vi "UpdateApp.vi"(7 "DefaultAppConfig? (f)":bool, 8 "ErrorArray In":errorcluster[](array[cluster]), 10 "clBusData in":T1={"BusNumber"=0, "EvtPluginINIFilePath"=path "", "EvtParams"=[], "EvtConfig"={"UTC Time 0"=timestamp(0 s since 1904-01-01), "Nominal Frequency"=60, "Reporting Rate"=60, "Fsamp"=960, "PosSeq"=FALSE}, "Start Time"=0.0, "End Time"=0.0, "PmuImpairPluginINIFilePath"=path "", "PmuImpairParams "=[["960"], ["8.19"], ["164"]], "PmuImpairConfig"={"FilterType"="", "bPosSeq"=TRUE}, "NetImpPluginINIFilePath"=path "", "NetImpParams"=[], "FlagImpPluginINIFilePath"=path "", "FlagImpParams"=[], "EvtReportArray"=[], "EventSignalArray"=[], "ImpairReportArray"=[], "NetworkTime"=[], "PktLoss"=[], "FlagImpArray"=[], "OutputToFilePluginINIFilePath"=path "", "Output File Path"=path "", "clConfigOptions"={"TIME_BASE"=1000000, "STN"="Bus_1", "IDCODE"=0, "rdoPolRect"=enum."Rectangular", "rdoFloatInt"=enum."Float", "PHUNIT"=1000000, "rdoFreqDfreq"=enum."Float", "CHNAM"=["VA", "VB", "VC", "V+", "IA", "IB", "IC", "I+"], "chkCfg2Prefix"=TRUE}, "AppPluginINIFilePath"=path "", "AppConfig"=variant, "AppOutput"=variant} {"clConfigOptions"."PHUNIT" max=16777216 step=1 format="%08d"; "clConfigOptions"."IDCODE" format="%02x"; "clConfigOptions"."TIME_BASE" max=16777216 step=1 format="%08d"; "ImpairReportArray"."Synx" format="%#_4g"; "EvtReportArray"."Synx" format="%#_4g"; "EvtConfig"."Reporting Rate" items=["10 FPS"=10, "12 FPS"=12, "15 FPS"=15, "20 FPS"=20, "25 FPS"=25, "30 FPS"=30, "50 FPS"=50, "60 FPS"=60]; "EvtConfig"."Nominal Frequency" items=["50 Hz"=50, "60 Hz"=60]}, 11 "Bus.lvclass":refnum<class "Bus.lvclass">) -> (0 "ErrorArray Out":errorcluster[](array[cluster]), 2 "clBusData out":T1={"BusNumber"=0, "EvtPluginINIFilePath"=path "", "EvtParams"=[], "EvtConfig"={"UTC Time 0"=timestamp(0 s since 1904-01-01), "Nominal Frequency"=60, "Reporting Rate"=60, "Fsamp"=960, "PosSeq"=FALSE}, "Start Time"=0.0, "End Time"=0.0, "PmuImpairPluginINIFilePath"=path "", "PmuImpairParams "=[["960"], ["8.19"], ["164"]], "PmuImpairConfig"={"FilterType"="", "bPosSeq"=TRUE}, "NetImpPluginINIFilePath"=path "", "NetImpParams"=[], "FlagImpPluginINIFilePath"=path "", "FlagImpParams"=[], "EvtReportArray"=[], "EventSignalArray"=[], "ImpairReportArray"=[], "NetworkTime"=[], "PktLoss"=[], "FlagImpArray"=[], "OutputToFilePluginINIFilePath"=path "", "Output File Path"=path "", "clConfigOptions"={"TIME_BASE"=1000000, "STN"="Bus_1", "IDCODE"=0, "rdoPolRect"=enum."Rectangular", "rdoFloatInt"=enum."Float", "PHUNIT"=1000000, "rdoFreqDfreq"=enum."Float", "CHNAM"=["VA", "VB", "VC", "V+", "IA", "IB", "IC", "I+"], "chkCfg2Prefix"=TRUE}, "AppPluginINIFilePath"=path "", "AppConfig"=variant, "AppOutput"=variant} {"clConfigOptions"."PHUNIT" max=16777216 step=1 format="%08d"; "clConfigOptions"."IDCODE" format="%02x"; "clConfigOptions"."TIME_BASE" max=16777216 step=1 format="%08d"; "ImpairReportArray"."Synx" format="%#_4g"; "EvtReportArray"."Synx" format="%#_4g"; "EvtConfig"."Reporting Rate" items=["10 FPS"=10, "12 FPS"=12, "15 FPS"=15, "20 FPS"=20, "25 FPS"=25, "30 FPS"=30, "50 FPS"=50, "60 FPS"=60]; "EvtConfig"."Nominal Frequency" items=["50 Hz"=50, "60 Hz"=60]}, 3 "Bus.lvclass":refnum<class "Bus.lvclass">)   [LabVIEW 2017, in "Bus_class.lvlib" / "Bus.lvclass"]
uses:
  Bus.lvclass
  TypeDefs/clBusData.ctl
  FrontPanel/TypeDefs/clEventConfig.ctl
  Modules/PmuImpairPlugins/PmuImpairPluginBase_class/TypeDefs/clImpairConfig.ctl
  Modules/EventPlugins/EventPluginBaseClass/TypeDefs/clEvtReportArray.ctl
  Modules/EventPlugins/EventPluginBaseClass/TypeDefs/clEvtReport.ctl
  Modules/EventPlugins/EventPluginBaseClass/TypeDefs/dblEvtSignalArray.ctl
  Modules/NetworkImpairmentModule/PublicAPI/Arguments/Broadcasts/dblNetworkTime.ctl
  Modules/NetworkImpairmentModule/PublicAPI/Arguments/Broadcasts/dblPktLoss.ctl
  Modules/FlagImpairModule/PublicAPI/Arguments/Broadcasts/ui32FlagImpairmentArray.ctl
  Modules/OutputToFilePlugins/OutputToFileBasePlugin/Typedefs/PmuCfgOpt.ctl
  <vilib>/Utility/error.llb/Error Cluster From Error Code.vi
  <vilib>/ErrorRing/Error Ring.xnode
  <vilib>/Utility/config.llb/NI_LVConfig.lvlib
  <userlib>/NIST/NISTErrorLib/NISTErrorLib.lvlib
  Framework.lvlib
  Modules/PmuImpairPlugins/PmuImpairPluginBase_class/PmuImpairPluginBase.lvclass
  Modules/EventPlugins/EventPluginBaseClass/EventPluginBaseClass.lvclass
  Modules/NetworkImpairmentModule/NetworkImpairmentModule.lvlib
  Modules/FlagImpairModule/FlagImpairModule.lvlib
  Modules/OutputToFilePlugins/OutputToFileBasePlugin/OutputToFileBasePlugin.lvclass
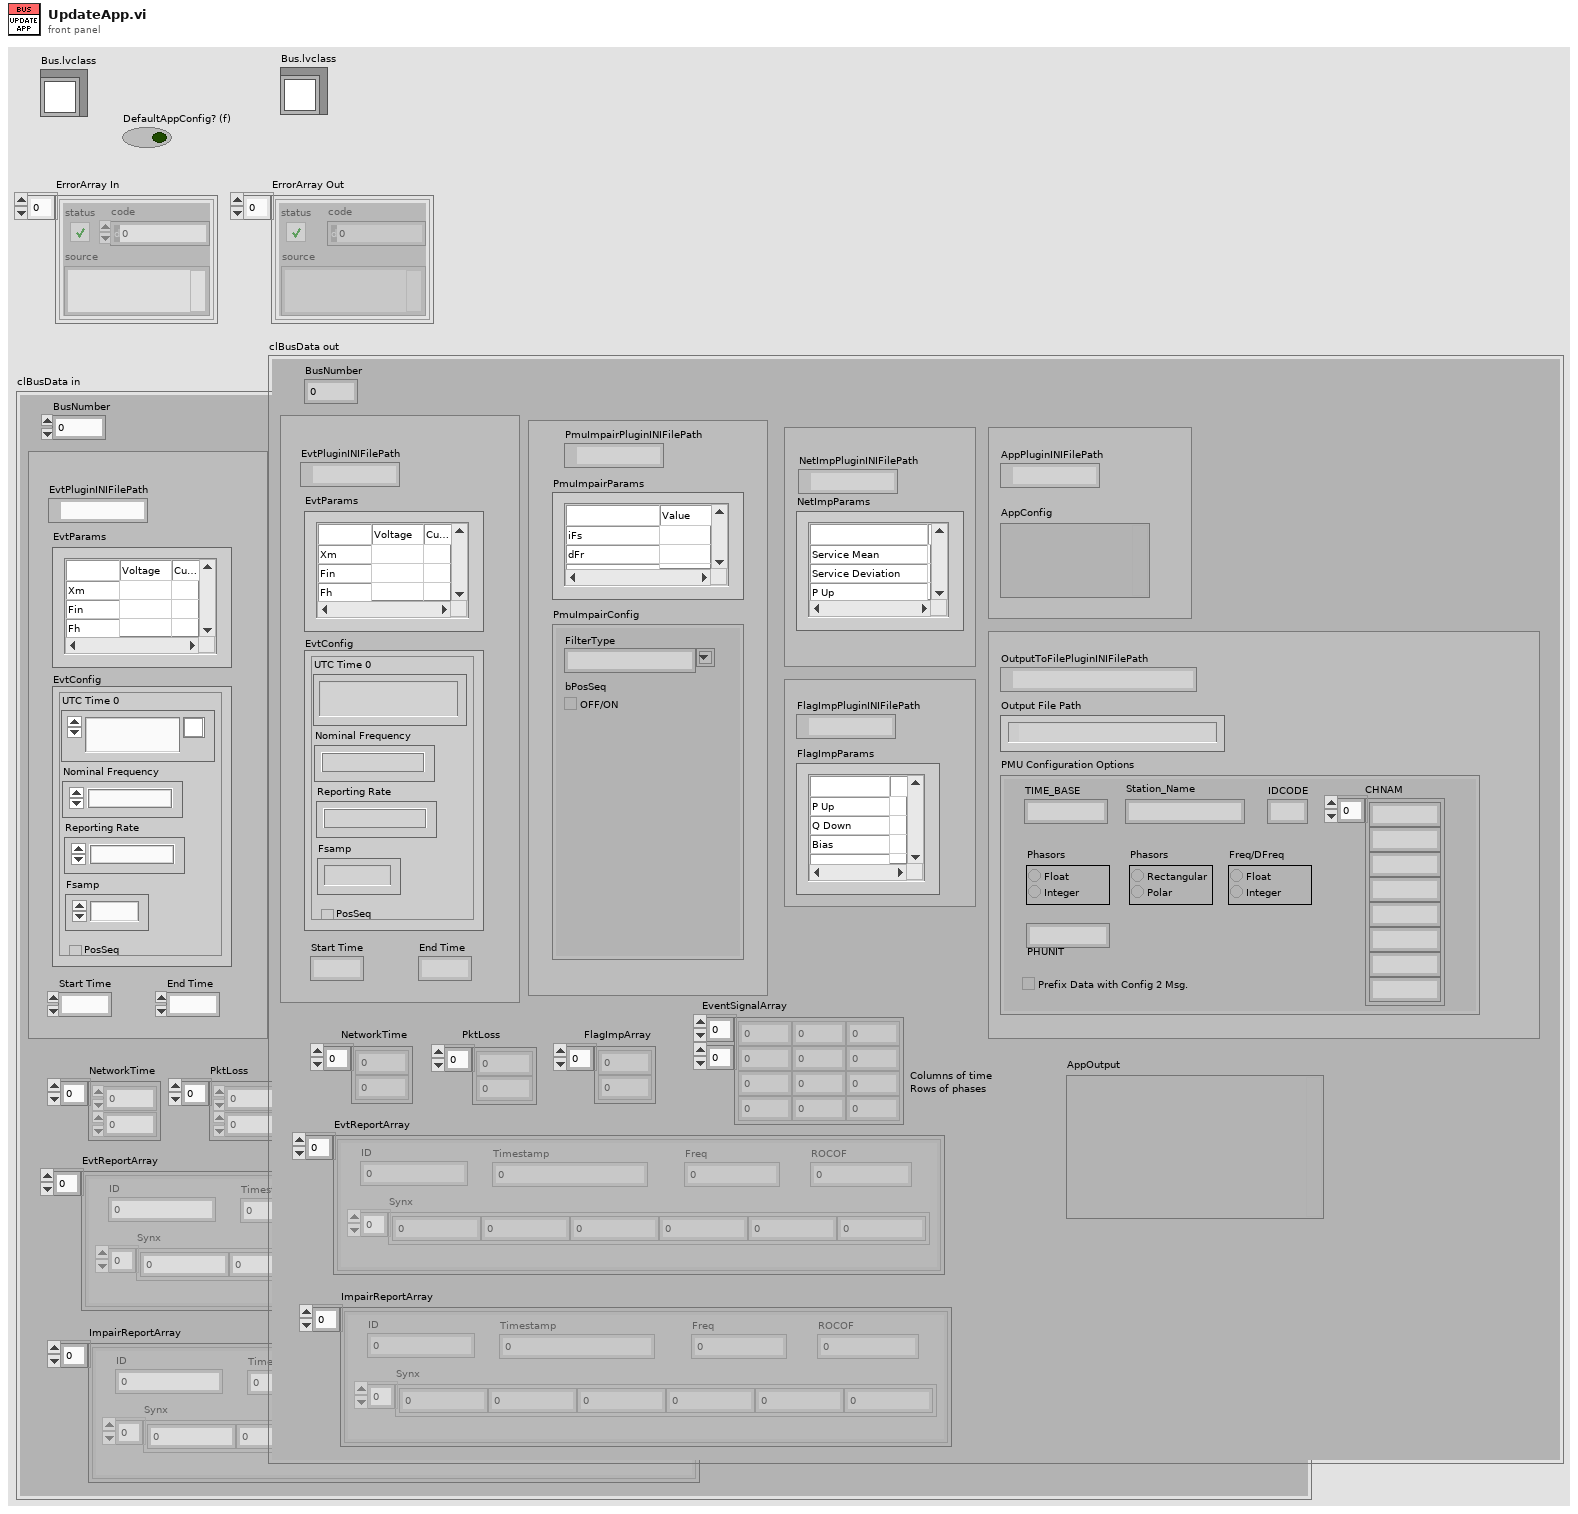
[diagram p1: front panel]
types:
  T1 = typedef "Bus_class.lvlib/Bus.lvclass/clBusData.ctl" = cluster{"BusNumber":u8, "EvtPluginINIFilePath":path, "EvtParams":string[][], "EvtConfig":T2, "Start Time":dbl, "End Time":dbl, "PmuImpairPluginINIFilePath":path, "PmuImpairParams ":string[][], "PmuImpairConfig":T3, "NetImpPluginINIFilePath":path, "NetImpParams":string[][], "FlagImpPluginINIFilePath":path, "FlagImpParams":string[][], "EvtReportArray":T4, "EventSignalArray":T6, "ImpairReportArray":T4, "NetworkTime":T7, "PktLoss":T8, "FlagImpArray":T9, "OutputToFilePluginINIFilePath":path, "Output File Path":path, "clConfigOptions":T10, "AppPluginINIFilePath":path, "AppConfig":variant, "AppOutput":variant}
  T2 = typedef "Framework.lvlib/clEventConfig.ctl" = cluster{"UTC Time 0":timestamp, "Nominal Frequency":u16, "Reporting Rate":u16, "Fsamp":u32, "PosSeq":bool}
  T3 = typedef "PmuImpairPlugins.lvlib/PmuImpairPluginBase.lvclass/clImpairConfig.ctl" = cluster{"FilterType":string, "bPosSeq":bool}
  T4 = typedef "EventPlugins.lvlib/EventPluginBaseClass.lvclass/clEvtReportArray.ctl" = T5[]
  T5 = typedef "EventPlugins.lvlib/EventPluginBaseClass.lvclass/clEvtReport.ctl" = cluster{"Timestamp":dbl, "Synx":cdb[], "Freq":dbl, "ROCOF":dbl, "ID":i16}
  T6 = typedef "EventPlugins.lvlib/EventPluginBaseClass.lvclass/dblEvtSignalArray.ctl" = dbl[][]
  T7 = typedef "NetworkImpairmentModule.lvlib/dblNetworkTime.ctl" = dbl[]
  T8 = typedef "NetworkImpairmentModule.lvlib/dblPktLoss.ctl" = dbl[]
  T9 = typedef "FlagImpairModule.lvlib/ui32FlagImpairmentArray.ctl" = u32[]
  T10 = typedef "OutputToFilePlugins.lvlib/OutputToFileBasePlugin.lvclass/PmuCfgOpt.ctl" = cluster{"TIME_BASE":u64, "STN":string, "IDCODE":u16, "rdoPolRect":enum32{"Rectangular", "Polar"}, "rdoFloatInt":enum32{"Float", "Integer"}, "PHUNIT":u64, "rdoFreqDfreq":enum32{"Float", "Integer"}, "CHNAM":string[], "chkCfg2Prefix":bool}
  T11 = typedef "Framework.lvlib/clFrameworkData.ctl" = cluster{"EvtINIFilePaths":path[], "BusClassInstances":refnum<class "Bus.lvclass">[], "PmuImpairINIFilePaths":path[], "FlagImpairINIFilePaths":path[], "NetImpairINIFilePaths":path[], "OutputToFileINIFilePaths":path[], "AppINIFilePaths":path[], "AppModuleID":i32, "OutputToFileID":i32}
  T12 = typedef "NI_LVConfig.lvlib/Config Data RefNum.ctl" = refnum<k1>
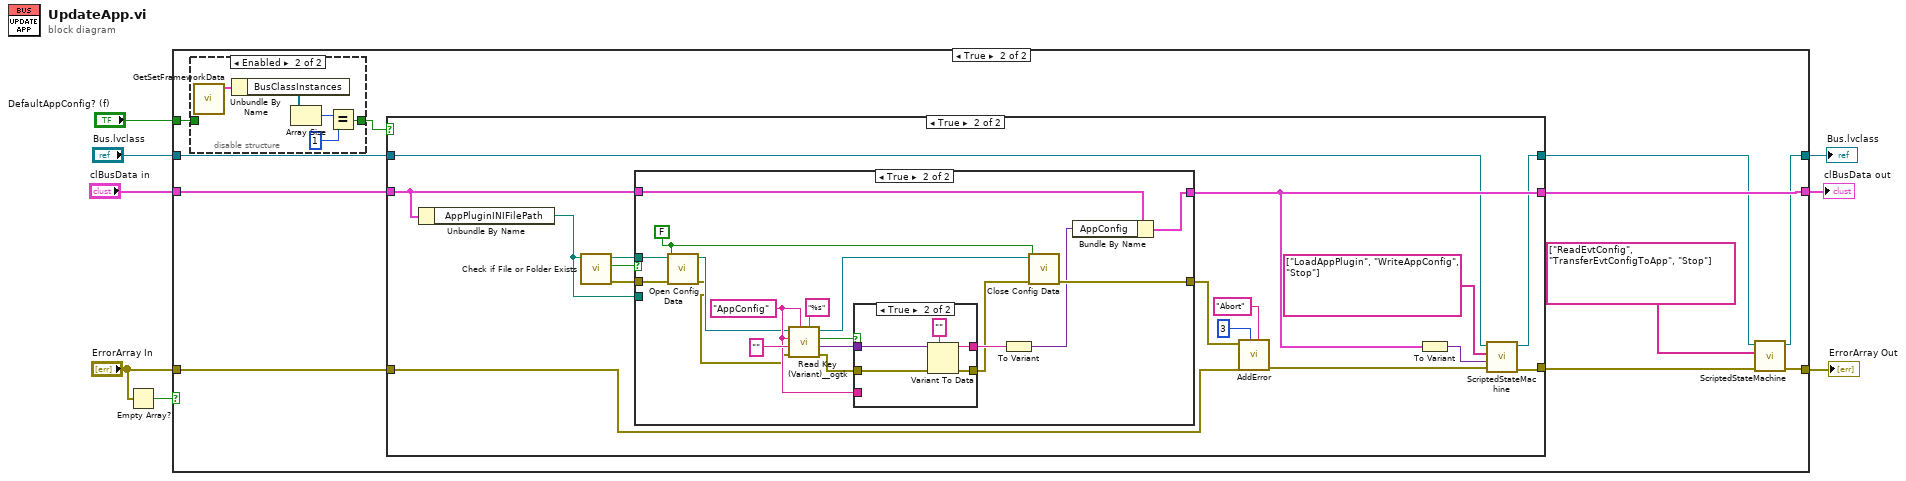
[diagram p0: block diagram]
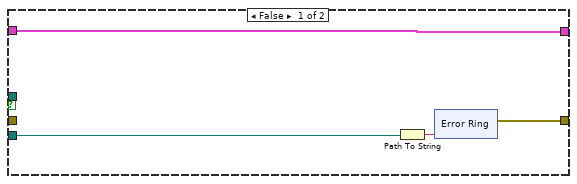
[diagram p5: hidden frame]
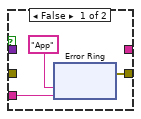
[diagram p6: hidden frame]
diagram:
  n1 = Empty Array?(array="ErrorArray In") -> (empty?=w5:bool)
  n2 = case shown="True" w5 {
    tunnel: "ErrorArray In" -> [w9 w20]
    tunnel: [w9 w17] -> w8
    tunnel: "Bus.lvclass" -> [w11 w16]
    tunnel: [w11 w14] -> w6
    tunnel: "clBusData in" -> [w10 w22]
    tunnel: [w10 w21] -> w2
    tunnel: "DefaultAppConfig? (f)" -> [_ w13]
    frame False {
    }
    frame True {
      n3 = disable-structure shown="Enabled" {
        disable-tunnel: [w23 w24] -> w12
        disable-tunnel: w13 -> [w23 _]
        frame Disabled {
        }
        frame Enabled {
          n4 = call "GetSetFrameworkData.vi"() -> ("clFrameworkData Out"=w25:T11)  [unwired: 11 in]
          n5 = Unbundle By Name(w25) -> ("BusClassInstances"=w26:refnum<class "Bus.lvclass">[])
          n6 = Array Size(array=w26) -> (size(s)=w27:i32)
          n7 = Equal?(x=w27, y=1) -> (x = y?=w24:bool)
        }
      }
      n8 = case shown="True" w12 {
        tunnel: w22 -> [w31 w38]
        tunnel: [w31 w37] -> w21
        tunnel: w20 -> [w30 w32]
        tunnel: [w30 w35] -> w19
        tunnel: w16 -> [w29 w34]
        tunnel: [w29 w33] -> w15
        frame False {
        }
        frame True {
          n9 = Unbundle By Name(w38) -> ("AppPluginINIFilePath"=w41:path)
          n10 = call <vilib>:"Check if File or Folder Exists.vi"("path"=w41) -> ("error out"=w45:errorcluster, "file or folder exists?"=w47:bool, "dup path"=w46:path)  [unwired: 8 in]
          n11 = case shown="True" w47 {
            tunnel: w46 -> [_ w76]
            tunnel: w45 -> [_ w75]
            tunnel: [w51 w73] -> w44
            tunnel: w41 -> [w49 _]
            tunnel: w38 -> [w48 w72]
            tunnel: [w48 w70] -> w37
            frame False {
              n12 = Path To String(path=w49) -> (string=w50:string)
              n13 = xnode "Error Ring"("parameter 0"=w50) -> ("error out"=w51:errorcluster)
            }
            frame True {
              w64 = "AppConfig" ("section")
              w74 = FALSE ("create file if necessary (T)")
              n14 = call <vilib>:"Open Config Data.vi"("error in (no error)"=w75, "create file if necessary (T)"=w74, "configuration file path"=w76) -> ("error out"=w61:errorcluster, "refnum"=w62:T12)  [unwired: 6 in, 1 out]
              n15 = call <userlib>:"Read Key (Variant)__ogtk.vi"("format string (%;%f)"="%s" ("float number format"), "section"=w64, "error in (no error)"=w61, "type"="", "key (optional)"=w64, "refnum"=w62) -> ("error out"=w66:errorcluster, "key-value"=w67:variant, "found?"=w65:bool, "refnum out"=w59:T12)  [unwired: 2 in]
              n16 = case shown="True" w65 {
                tunnel: w67 -> [_ w92]
                tunnel: w66 -> [_ w91]
                tunnel: [_ w89] -> w63
                tunnel: [w79 w88] -> w60
                tunnel: w64 -> [w77 _]
                frame False {
                  n17 = xnode "Error Ring"("parameter 0"="App", "parameter 1"=w77) -> ("error out"=w79:errorcluster)
                }
                frame True {
                  n18 = Variant To Data(error in=w91, type="", Variant=w92) -> (data=w89:string, error out=w88:errorcluster)
                }
              }
              n19 = To Variant(anything=w63) -> (Variant=w71:variant)
              n20 = call <vilib>:"Close Config Data.vi"("error in (no error)"=w60, "write file if changed (T)"=w74, "refnum"=w59) -> ("error out"=w73:errorcluster)  [unwired: 7 in, 1 out]
              n21 = Bundle By Name(cluster=w72, "AppConfig"=w71) -> (w70:T1)
            }
          }
          n22 = call <userlib>:"AddError.vi"("Severity"="Abort", "Priority"=u8 3, "ErrorArray"=w32, "error in (no error)"=w44) -> ("ErrorArray"=w36:errorcluster[])  [unwired: 6 in, 1 out]
          n23 = To Variant(anything=w37) -> (Variant=w39:variant)
          n24 = call "ScriptedStateMachine.vi"("ErrorArray In"=w36, "Data in"=w39, "Script"=string[] ["LoadAppPlugin", "WriteAppConfig", "Stop"], "Bus"=w34) -> ("ErrorArray Out"=w35:errorcluster[], "Bus"=w33:refnum<class "Bus.lvclass">)  [unwired: 5 in, 1 out]
        }
      }
      n25 = call "ScriptedStateMachine.vi"("ErrorArray In"=w19, "Script"=string[] ["ReadEvtConfig", "TransferEvtConfigToApp", "Stop"], "Bus"=w15) -> ("ErrorArray Out"=w17:errorcluster[], "Bus"=w14:refnum<class "Bus.lvclass">)  [unwired: 6 in, 1 out]
    }
  }
  "Bus.lvclass" <- w6
  "ErrorArray Out" <- w8
  "clBusData out" <- w2
